vi "picture plot.vi"(8 "error in":errorcluster) -> (0 "error out":errorcluster, 3 "Images":picture[](array[picture]))   [LabVIEW 2018]
uses:
  channel_cluster.ctl
  <vilib>/picture/cartesn2.llb/XY Plot Type.ctl
  CAEN globals.vi
panel:
  out "new picture":picture
  # "mrd1\nmrd2\ntank\nveto\nother\nmaster"
  # "mrd1 = pink\nmrd2 = green\ntank = blue\nveto = orange\nmasters = purple\nother = red"
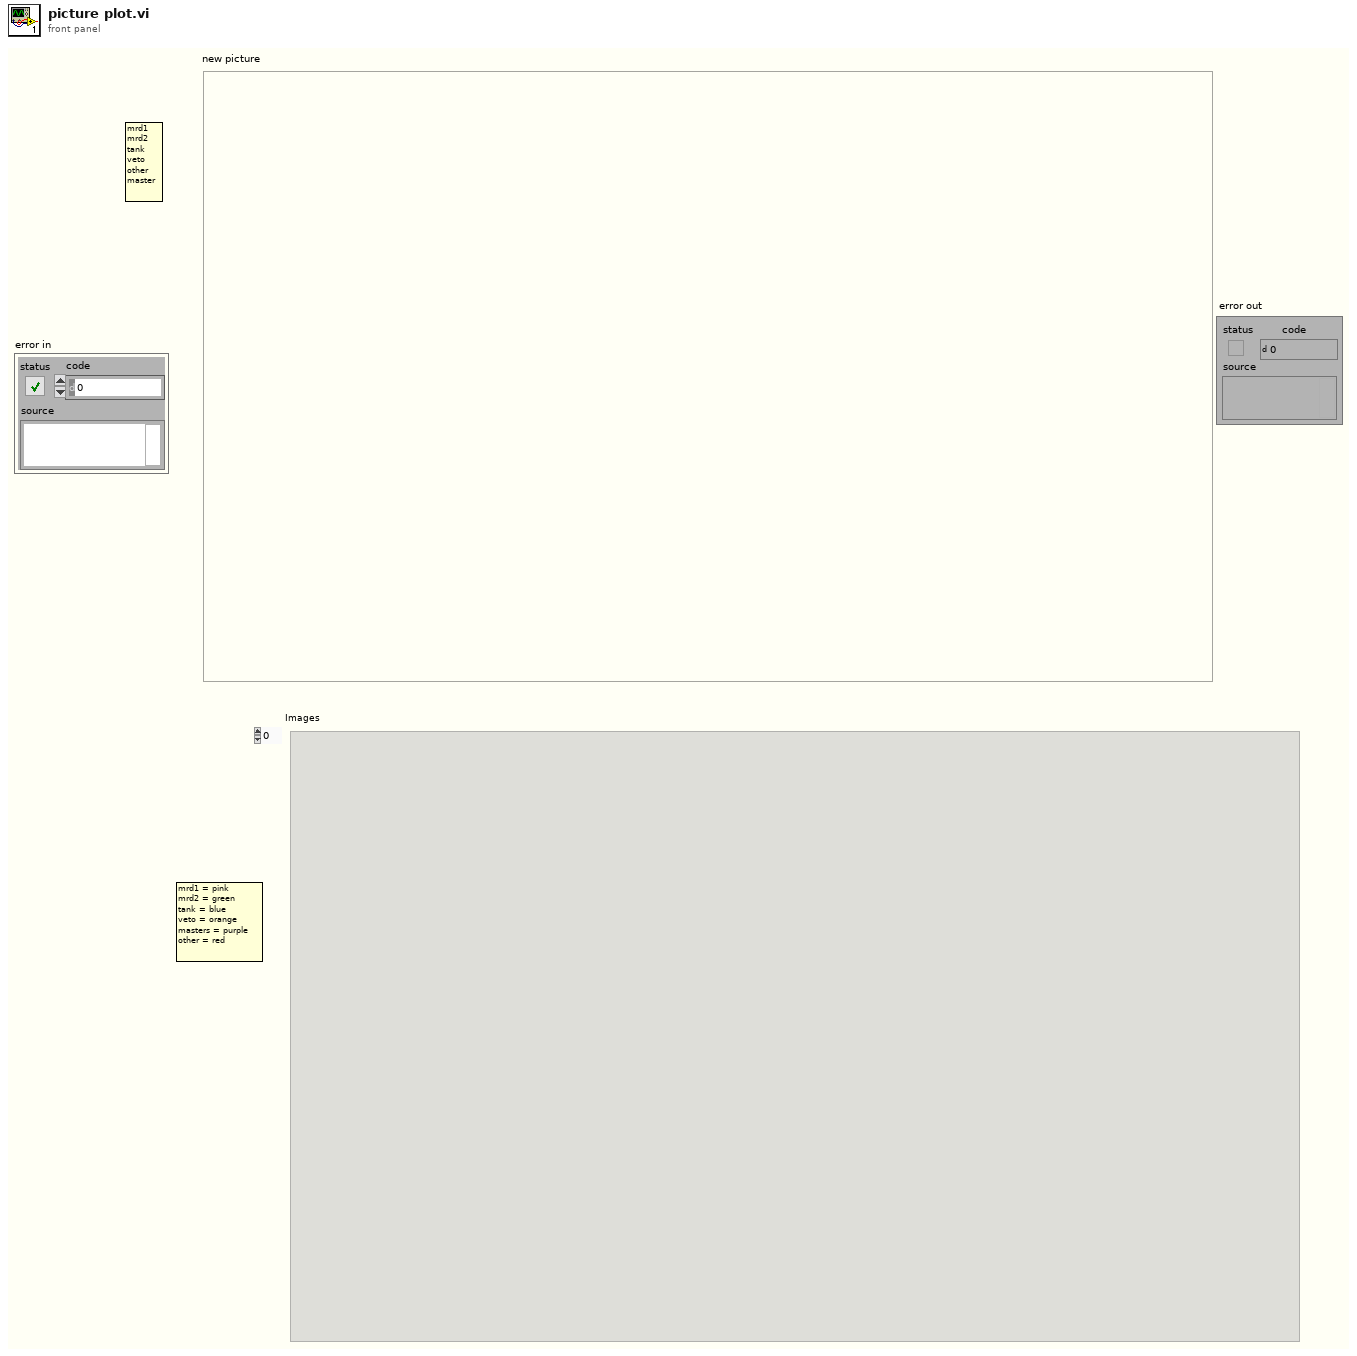
[diagram p1: front panel]
types:
  T1 = typedef "channel_cluster.ctl" = cluster{"Channel Name":string, "Crate":i32, "Card Type":string, "Card":i32, "Channel":i32, "Status Icon":picture, "Vmon (V)":dbl, "Vset (V)":dbl, "Imon (A)":dbl, "Iset (A)":dbl, "Timestamp":string, "ON/OFF":bool, "Status":string, "Vswmax (V)":dbl, "Flag":bool, "Vfile (V)":dbl, "Error Logged":bool[], "enable_file":bool}
  T2 = cluster{"x minimum":dbl, "x maximum":dbl, "x log?":bool, "x precision":u8, "x format":enum8{"Decimal", "Scientific", "Engineering", "Binary", "Octal", "Hex", "Timestamp"}, "y minimum":dbl, "y maximum":dbl, "y log?":bool, "y precision":u8, "y format":enum8{"Decimal", "Scientific", "Engineering", "Binary", "Octal", "Hex", "Timestamp"}}
  T3 = cluster{"Width":u16, "Style":enum32{"Solid", "Dash", "Dot", "DashDot", "DashDotDot"}}[]
  T4 = enum8{"Decimal", "Scientific", "Engineering", "Binary", "Octal", "Hex", "Timestamp"}
  T5 = typedef "XY Plot Type.ctl" = enum16{"points", "squares", "circles", "connected points", "connected squares", "connected circles", "comb plot", "sized scatter plot", "sized-colored scatter plot", "min-max lines"}
  T6 = cluster{"plot color":u32, "XY plot type":T5, "baseline":dbl}
  T7 = cluster{"line color":u32, "text color":u32, "tick length(3)":i16, "crossing axes":bool, "visible grid?":bool}
  T8 = cluster{"plot color":u32, "XY plot type":T5, "baseline":dbl}[]
  T9 = typedef "imagedata.ctl" = cluster{"image type":i32, "image depth":i32, "image":u8[], "mask":u8[], "colors":u32[], "Rectangle":cluster{"left":i16, "top":i16, "right":i16, "bottom":i16}}
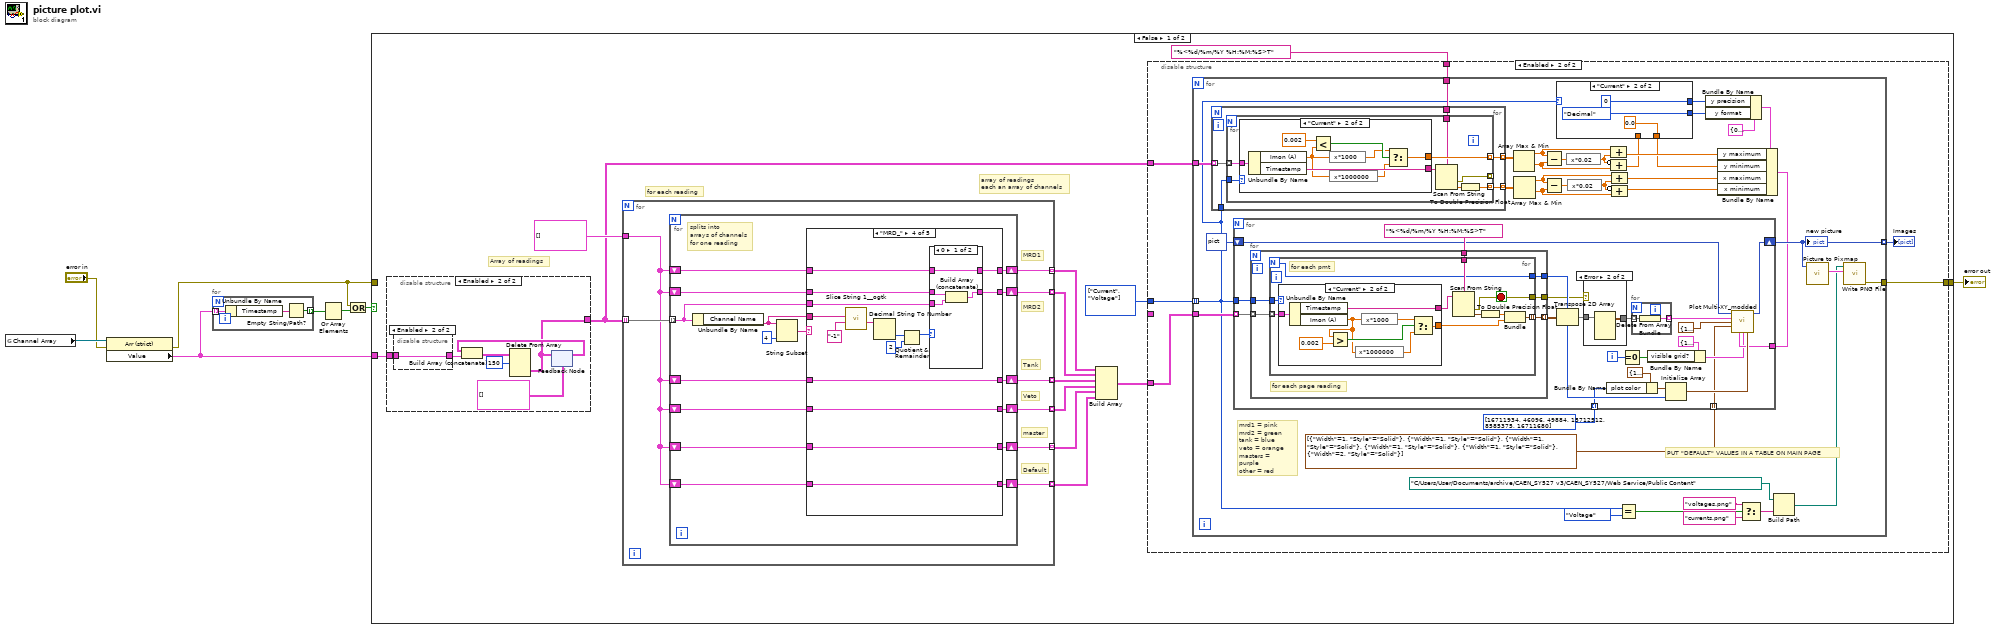
[diagram p0: block diagram]
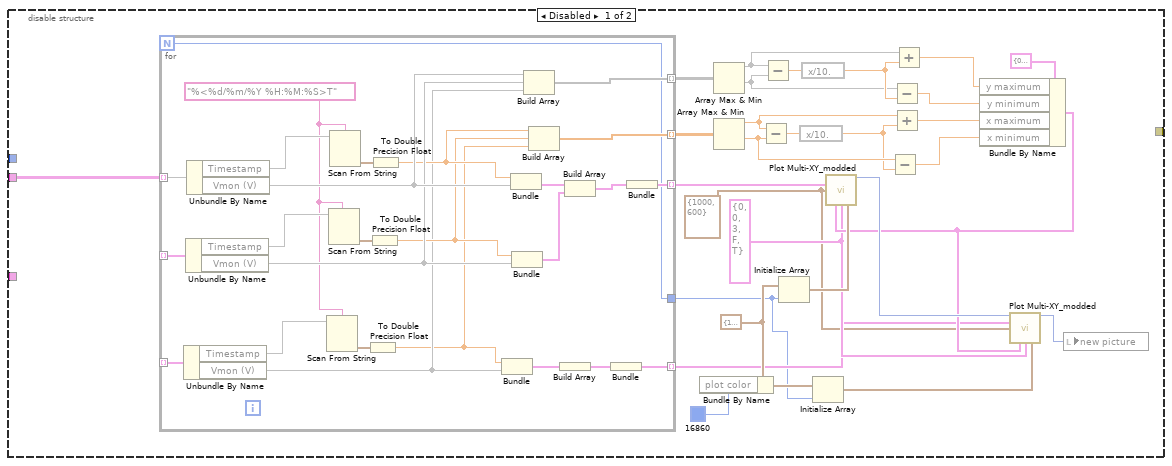
[diagram p4: hidden frame]
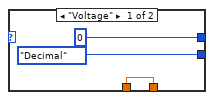
[diagram p5: hidden frame]
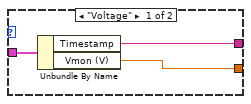
[diagram p7: hidden frame]
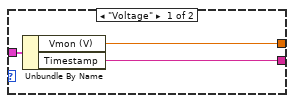
[diagram p8: hidden frame]
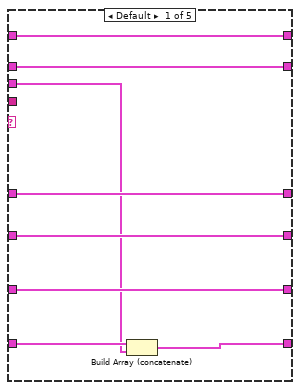
[diagram p9: hidden frame]
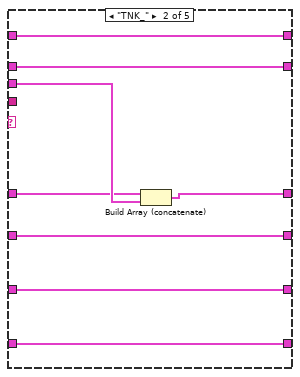
[diagram p10: hidden frame]
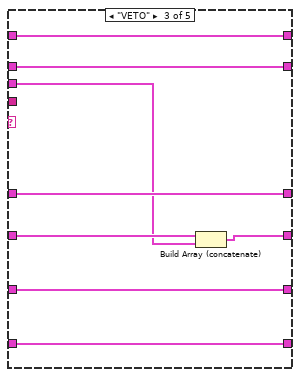
[diagram p11: hidden frame]
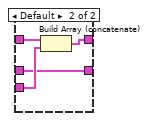
[diagram p12: hidden frame]
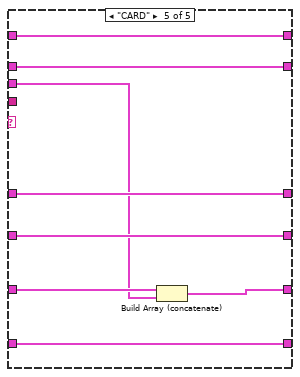
[diagram p13: hidden frame]
diagram:
  n1 = global read "CAEN globals.vi" "Channel Array"() -> (w7:refnum<vi>)
  n2 = property class="Arr (strict)"(reference=w7, error in="error in") -> (error out=w3:errorcluster, "Value"=w5:T1[])  [unwired: 1 out]
  n3 = for {
    tunnel: w5 -> [w11] mode=indexing
    tunnel: [w9] -> w4 mode=indexing
    n4 = Unbundle By Name(w11) -> ("Timestamp"=w10:string)
    n5 = Empty String/Path?(string/path=w10) -> (empty?=w9:bool)
  }
  n6 = Or Array Elements(Boolean array=w4) -> (logical OR=w2:bool)
  n7 = Or(x=w3, y=w2) -> (x .or. y?=w1:bool)
  n8 = case shown="False" w1 {
    tunnel: [w15 w294] -> w8
    tunnel: w5 -> [w12 _]
    tunnel: w3 -> [_ w294]
    frame False {
      w14 = enum16{"Current", "Voltage"}[] [enum."Current", enum."Voltage"] items=["Current", "Voltage"]
      # "array of readings\neach an array of channels"
      # "for each reading"
      # "Array of readings"
      n9 = disable-structure shown="Enabled" {
        disable-tunnel: [_ w27] -> w18
        disable-tunnel: w12 -> [_ w25]
        frame Disabled {
        }
        frame Enabled {
          n10 = disable-structure shown="Enabled" {
            disable-tunnel: [_ w32] -> w29
            disable-tunnel: w25 -> [_ w32]
            frame Disabled {
            }
            frame Enabled {
            }
          }
          n11 = feedback #1(T1[][] [] ("appended array")) -> (w30:T1[][])
          n12 = Build Array (concatenate)(w30, w29) -> (w28:T1[][])
          n13 = Delete From Array(array=w28, length=150) -> (deleted portion=w27:T1[][])  [unwired: 2 in, 1 out]
          n14 = feedback-in #1(w27) -> ()
        }
      }
      n15 = for {
        tunnel: w18 -> [w222] mode=indexing
        tunnel: [w221] -> w19 mode=indexing
        tunnel: [w220] -> w23 mode=indexing
        tunnel: [w219] -> w16 mode=indexing
        tunnel: [w218] -> w22 mode=indexing
        tunnel: [w217] -> w21 mode=indexing
        tunnel: T1[] [] -> [w216]
        tunnel: [w215] -> w13 mode=indexing
        # "master"
        # "Default"
        # "Veto"
        # "Tank"
        # "MRD2"
        # "MRD1"
        n16 = for {
          shift-right: [w232] -> w218
          shift-left: w216 -> [w231]
          shift-right: [w234] -> w219
          shift-left: w216 -> [w233]
          shift-right: [w228] -> w220
          shift-left: w216 -> [w235]
          shift-right: [w229] -> w221
          shift-left: w216 -> [w236]
          tunnel: w222 -> [w230] mode=indexing
          shift-right: [w227] -> w217
          shift-left: w216 -> [w226]
          shift-right: [w223] -> w215
          shift-left: w216 -> [w224]
          # "splits into \narrays of channels\nfor one reading"
          n17 = Unbundle By Name(w230) -> ("Channel Name"=w225:string)
          n18 = String Subset(string=w225, length (rest)=4 ("length (rest)")) -> (substring=w237:string)  [unwired: 1 in]
          n19 = case shown="\"MRD_\"" w237 {
            tunnel: w236 -> [w246 w254 w262 w272 w293]
            tunnel: w235 -> [w245 w253 w261 w268 w292]
            tunnel: [w244 w250 w260 w274 w291] -> w234
            tunnel: w233 -> [w244 w251 w260 w274 w291]
            tunnel: [w243 w249 w257 w273 w290] -> w232
            tunnel: w231 -> [w243 w249 w259 w273 w290]
            tunnel: w230 -> [w239 w252 w258 w271 w288]
            tunnel: [w246 w254 w262 w270 w293] -> w229
            tunnel: [w245 w253 w261 w269 w292] -> w228
            tunnel: [w242 w248 w256 w267 w287] -> w227
            tunnel: w226 -> [w242 w248 w256 w267 w289]
            tunnel: w225 -> [_ _ _ w266 _]
            tunnel: w224 -> [w241 w247 w255 w263 w286]
            tunnel: [w240 w247 w255 w263 w286] -> w223
            frame Default {
              n20 = Build Array (concatenate)(w241, w239) -> (w240:T1[])
            }
            frame "TNK_" {
              n21 = Build Array (concatenate)(w251, w252) -> (w250:T1[])
            }
            frame "VETO" {
              n22 = Build Array (concatenate)(w259, w258) -> (w257:T1[])
            }
            frame "MRD_" {
              n23 = call <userlib>:"Slice String 1__ogtk.vi"("Subset (i:j)"="-1", "String"=w266) -> ("Substring (String[i:j])"=w277:string)  [unwired: 7 in]
              n24 = Decimal String To Number(string=w277) -> (number=w276:i32)  [unwired: 2 in, 1 out]
              n25 = Quotient & Remainder(x=w276, y=2) -> (x-y*floor(x/y)=w265:i32)  [unwired: 1 out]
              n26 = case shown="0" w265 {
                tunnel: w272 -> [w281 w285]
                tunnel: w271 -> [w278 w284]
                tunnel: [w281 w283] -> w270
                tunnel: [w279 w282] -> w269
                tunnel: w268 -> [w280 w282]
                frame 0 {
                  n27 = Build Array (concatenate)(w280, w278) -> (w279:T1[])
                }
                frame Default {
                  n28 = Build Array (concatenate)(w285, w284) -> (w283:T1[])
                }
              }
            }
            frame "CARD" {
              n29 = Build Array (concatenate)(w289, w288) -> (w287:T1[])
            }
          }
        }
      }
      n30 = Build Array(w19, w23, w16, w22, w21, w13) -> (w20:T1[][][])
      n31 = disable-structure shown="Enabled" {
        disable-tunnel: _ -> [w34 _]
        disable-tunnel: w20 -> [_ w91]
        disable-tunnel: w18 -> [_ w93]
        disable-tunnel: "%<%d/%m/%Y %H:%M:%S>T" ("format string") -> [_ w92]
        disable-tunnel: [_ w90] -> w15
        disable-tunnel: w14 -> [_ w88]
        frame Disabled {
          w41 = T6 {"plot color"=16711680, "XY plot type"=enum."connected points", "baseline"=0.0} ("xy plot cosmetics")
          w42 = T7 {"line color"=0, "text color"=0, "tick length(3)"=3, "crossing axes"=FALSE, "visible grid?"=TRUE} ("cartesian grid cosmetics")
          w38 = cluster{"width":i16, "height":i16} {"width"=1000, "height"=600} ("dimensions (w,h)")
          n32 = for {
            N -> [w75]
            tunnel: w34 -> [w87] mode=indexing
            tunnel: [w82] -> w61 mode=indexing
            tunnel: [w76] -> w60 mode=indexing
            tunnel: [w77] -> w54 mode=indexing
            tunnel: _ -> [w79] mode=indexing
            tunnel: [w75] -> w35
            tunnel: _ -> [w68] mode=indexing
            tunnel: [w64] -> w39 mode=indexing
            w67 = "%<%d/%m/%Y %H:%M:%S>T" ("format string")
            n33 = Unbundle By Name(w68) -> ("Timestamp"=w70, "Vmon (V)"=w63)
            n34 = Unbundle By Name(w79) -> ("Timestamp"=w80, "Vmon (V)"=w73)
            n35 = Unbundle By Name(w87) -> ("Timestamp"=w86, "Vmon (V)"=w74)
            n36 = Scan From String(format string=w67, input string=w70) -> (output 1=w69:timestamp)  [unwired: 3 in, 3 out]
            n37 = Scan From String(format string=w67, input string=w80) -> (output 1=w81:timestamp)  [unwired: 3 in, 3 out]
            n38 = Scan From String(format string=w67, input string=w86) -> (output 1=w85:timestamp)  [unwired: 3 in, 3 out]
            n39 = To Double Precision Float(number=w69) -> (double precision float=w62:dbl)
            n40 = To Double Precision Float(number=w81) -> (double precision float=w71:dbl)
            n41 = To Double Precision Float(number=w85) -> (double precision float=w72:dbl)
            n42 = Bundle(w62, "Vmon (V)"=w63) -> (w66:cluster{dbl, "Vmon (V)":void})  [unwired: 1 in]
            n43 = Bundle(w72, "Vmon (V)"=w74) -> (w84:cluster{dbl, "Vmon (V)":void})  [unwired: 1 in]
            n44 = Bundle(w71, "Vmon (V)"=w73) -> (w78:cluster{dbl, "Vmon (V)":void})  [unwired: 1 in]
            n45 = Build Array(w74, w73, w63) -> (w77:void[])
            n46 = Build Array(w72, w71, w62) -> (w76:dbl[])
            n47 = Build Array(w66) -> (w65:cluster{dbl, "Vmon (V)":void}[])
            n48 = Build Array(w84, w78) -> (w83:cluster{dbl, "Vmon (V)":void}[])
            n49 = Bundle(w65) -> (w64:cluster{cluster{dbl, "Vmon (V)":void}[]})  [unwired: 1 in]
            n50 = Bundle(w83) -> (w82:cluster{cluster{dbl, "Vmon (V)":void}[]})  [unwired: 1 in]
          }
          n51 = Bundle By Name(cluster=w41, "plot color"=u32 16860) -> (w37:T6)
          n52 = Array Max & Min(array=w54) -> (max value=w49, min value=w48)  [unwired: 2 out]
          n53 = Array Max & Min(array=w60) -> (max value=w58:dbl, min value=w57:dbl)  [unwired: 2 out]
          n54 = Subtract(x=w58, y=w57) -> (x-y=w59:dbl)
          n55 = Subtract(x=w49, y=w48) -> (x-y=w50:dbl)
          n56 = Initialize Array(w41, w35) -> (w45:T8)
          n57 = expression code="x/10."(w59) -> (w56:dbl)
          n58 = expression code="x/10."(w50) -> (w51:dbl)
          n59 = Initialize Array(w37, w35) -> (w36:T8)
          n60 = Subtract(x=w57, y=w56) -> (x-y=w52:dbl)
          n61 = Subtract(x=w48, y=w51) -> (x-y=w46:dbl)
          n62 = Add(x=w58, y=w56) -> (x+y=w53:dbl)
          n63 = Add(x=w49, y=w51) -> (x+y=w47:dbl)
          n64 = Bundle By Name(cluster=T2 {"x minimum"=0.0, "x maximum"=0.0, "x log?"=FALSE, "x precision"=2, "x format"=enum."Timestamp", "y minimum"=0.0, "y maximum"=0.0, "y log?"=FALSE, "y precision"=0, "y format"=enum."Decimal"} ("cartesian axis attributes"), "y maximum"=w47, "y minimum"=w46, "x maximum"=w53, "x minimum"=w52) -> (w43:T2)
          n65 = call "Plot Multi-XY_modded.vi"("data"=w61, "dimensions (w,h)"=w38, "cartesian axis attributes"=w43, "cartesian grid cosmetics"=w42, "XY plot cosmetics"=w45) -> ("new picture"=w44:picture)  [unwired: 10 in]
          n66 = call "Plot Multi-XY_modded.vi"("picture"=w44, "data"=w39, "dimensions (w,h)"=w38, "cartesian axis attributes"=w43, "cartesian grid cosmetics"=w42, "XY plot cosmetics"=w36) -> ("new picture"=w33:picture)  [unwired: 9 in]
          n67 = local write "new picture"(w33) -> ()
        }
        frame Enabled {
          n68 = for {
            tunnel: w93 -> [w124]
            tunnel: w92 -> [w123]
            tunnel: w91 -> [w121]
            tunnel: [w117] -> w90
            tunnel: [w109] -> w89 mode=indexing
            tunnel: w88 -> [w105] mode=indexing
            # "PUT \"DEFAULT\" VALUES IN A TABLE ON MAIN PAGE"
            # "mrd1 = pink\nmrd2 = green\ntank = blue\nveto = orange\nmasters = purple\nother = red"
            n69 = for {
              tunnel: w124 -> [w195] mode=indexing
              tunnel: [w194] -> w96 mode=indexing
              tunnel: w123 -> [w193]
              tunnel: [w192] -> w122 mode=indexing
              tunnel: w105 -> [w191]
              n70 = for {
                tunnel: w195 -> [w203] mode=indexing
                tunnel: [w202] -> w194 mode=indexing
                tunnel: w193 -> [w199]
                tunnel: [w198] -> w192 mode=indexing
                tunnel: w191 -> [w197]
                tunnel: [w196] -> _ mode=indexing
                n71 = case shown="\"Current\"" w197 {
                  tunnel: w203 -> [w206 w214]
                  tunnel: [w205 w211] -> w202
                  tunnel: [w204 w213] -> w200
                  frame "Voltage" {
                    n72 = Unbundle By Name(w206) -> ("Vmon (V)"=w205:dbl, "Timestamp"=w204:string)
                  }
                  frame "Current" {
                    n73 = Unbundle By Name(w214) -> ("Imon (A)"=w210:dbl, "Timestamp"=w213:string)
                    n74 = Less?(x=0.002, y=w210) -> (x < y?=w209:bool)
                    n75 = expression code="x*1000"(w210) -> (w208:dbl)
                    n76 = expression code="x*1000000"(w210) -> (w207:dbl)
                    n77 = Select(t=w208, s=w209, f=w207) -> (s? t:f=w211:dbl)
                  }
                }
                n78 = Scan From String(format string=w199, input string=w200) -> (error out=w196:errorcluster, output 1=w201:dbl)  [unwired: 3 in, 2 out]
                n79 = To Double Precision Float(number=w201) -> (double precision float=w198:dbl)
              }
            }
            n80 = Array Max & Min(array=w96) -> (max value=w99:dbl, min value=w100:dbl)  [unwired: 2 out]
            n81 = Array Max & Min(array=w122) -> (max value=w129:dbl, min value=w128:dbl)  [unwired: 2 out]
            n82 = Subtract(x=w99, y=w100) -> (x-y=w98:dbl)
            n83 = Subtract(x=w129, y=w128) -> (x-y=w130:dbl)
            n84 = expression code="x*0.02"(w98) -> (w101:dbl)
            n85 = expression code="x*0.02"(w130) -> (w127:dbl)
            n86 = Compound Arithmetic op=ADD(w99, w101) -> (w97:dbl)
            n87 = Compound Arithmetic op=ADD(invert w101, w100) -> (w95:dbl)
            n88 = case shown="\"Current\"" w105 {
              tunnel: [u8 0 ("y precision") u8 0 ("y precision")] -> w104
              tunnel: [T4."Decimal" ("y format") T4."Decimal" ("y format")] -> w103
              tunnel: [w131 0.0] -> w94
              tunnel: w95 -> [w131 _]
              frame "Voltage" {
              }
              frame "Current" {
              }
            }
            n89 = Compound Arithmetic op=ADD(w129, w127) -> (w126:dbl)
            n90 = Compound Arithmetic op=ADD(invert w127, w128) -> (w125:dbl)
            n91 = Equal?(x=w105, y=enum16{"Current", "Voltage"}."Voltage") -> (x = y?=w111:bool)
            n92 = Bundle By Name(cluster=T2 {"x minimum"=0.0, "x maximum"=0.0, "x log?"=FALSE, "x precision"=2, "x format"=enum."Timestamp", "y minimum"=0.0, "y maximum"=0.0, "y log?"=FALSE, "y precision"=0, "y format"=enum."Decimal"} ("cartesian axis attributes"), "y precision"=w104, "y format"=w103) -> (w106:T2)
            n93 = Bundle By Name(cluster=w106, "y maximum"=w97, "y minimum"=w94, "x maximum"=w126, "x minimum"=w125) -> (w102:T2)
            n94 = for {
              tunnel: w102 -> [w157]
              tunnel: w121 -> [w143] mode=indexing
              tunnel: u32[] [16711934, 46096, 49884, 15712512, 8585375, 16711680] -> [w151] mode=indexing
              shift-right: [w150] -> w109
              shift-left: picture data[5B] ("new picture") -> [w149]
              tunnel: T3 [{"Width"=1, "Style"=enum."Solid"}, {"Width"=1, "Style"=enum."Solid"}, {"Width"=1, "Style"=enum."Solid"}, {"Width"=1, "Style"=enum."Solid"}, {"Width"=1, "Style"=enum."Solid"}, {"Width"=2, "Style"=enum."Solid"}] -> [w138] mode=indexing
              tunnel: w105 -> [w137]
              i -> [w140]
              n95 = for {
                tunnel: w143 -> [w169] mode=indexing
                tunnel: [w165] -> w155
                tunnel: "%<%d/%m/%Y %H:%M:%S>T" ("format string") -> [w168]
                tunnel: [w167] -> w145 mode=indexing
                tunnel: [w166] -> w144
                tunnel: w137 -> [w164]
                # "for each page reading"
                n96 = for {
                  N -> [w171]
                  tunnel: w169 -> [w179] mode=indexing
                  tunnel: [w174] -> w167 mode=indexing
                  tunnel: w168 -> [w173]
                  tunnel: [w172] -> w166
                  tunnel: [w171] -> w165
                  tunnel: w164 -> [w170]
                  stop <- w172 stop-if-true
                  # "for each pmt"
                  n97 = case shown="\"Current\"" w170 {
                    tunnel: w179 -> [w182 w190]
                    tunnel: [w181 w189] -> w178
                    tunnel: [w180 w184] -> w176
                    frame "Voltage" {
                      n98 = Unbundle By Name(w182) -> ("Timestamp"=w181:string, "Vmon (V)"=w180:dbl)
                    }
                    frame "Current" {
                      n99 = Unbundle By Name(w190) -> ("Timestamp"=w189:string, "Imon (A)"=w183:dbl)
                      n100 = Greater?(x=w183, y=0.002 ("x")) -> (0:w186:bool)
                      n101 = expression code="x*1000000"(w183) -> (w188:dbl)
                      n102 = expression code="x*1000"(w183) -> (w187:dbl)
                      n103 = Select(t=w187, s=w186, f=w188) -> (s? t:f=w184:dbl)
                    }
                  }
                  n104 = Scan From String(format string=w173, input string=w178) -> (error out=w172:errorcluster, output 1=w177:timestamp)  [unwired: 3 in, 2 out]
                  n105 = To Double Precision Float(number=w177) -> (double precision float=w175:dbl)
                  n106 = Bundle(w175, "Imon (A)"=w176) -> (w174:cluster{dbl, "Imon (A)":dbl})  [unwired: 1 in]
                }
              }
              n107 = Transpose 2D Array(2D array=w145) -> (transposed array=w148:cluster{dbl, "Imon (A)":dbl}[][])
              n108 = case shown="Error" w144 {
                tunnel: w148 -> [w159 w161]
                tunnel: [w159 w160] -> w147
                frame No Error {
                }
                frame Error {
                  n109 = Delete From Array(array=w161) -> (array with subset deleted=w160:cluster{dbl, "Imon (A)":dbl}[][])  [unwired: 3 in, 1 out]
                }
              }
              n110 = Bundle By Name(cluster=T6 {"plot color"=16711680, "XY plot type"=enum."connected circles", "baseline"=0.0} ("xy plot cosmetics"), "plot color"=w151) -> (w152:T6)
              n111 = Equal To 0?(x=w140) -> (x = 0?=w139:bool)
              n112 = for {
                tunnel: w147 -> [w163] mode=indexing
                tunnel: [w162] -> w146 mode=indexing
                n113 = Bundle(w163) -> (w162:cluster{cluster{dbl, "Imon (A)":dbl}[]})  [unwired: 1 in]
              }
              n114 = Bundle By Name(cluster=T7 {"line color"=13816530, "text color"=0, "tick length(3)"=3, "crossing axes"=FALSE, "visible grid?"=TRUE} ("cartesian grid cosmetics"), "visible grid?"=w139) -> (w141:T7)
              n115 = Initialize Array(w152, w155) -> (w158:T8)
              n116 = call "Plot Multi-XY_modded.vi"("picture"=w149, "data"=w146, "dimensions (w,h)"=cluster{"width":i16, "height":i16} {"width"=1000, "height"=600}, "line style"=w138, "cartesian axis attributes"=w157, "cartesian grid cosmetics"=w141, "XY plot cosmetics"=w158) -> ("new picture"=w150:picture)  [unwired: 8 in]
            }
            "new picture" <- w109
            n117 = Select(t="voltages.png" ("name or relative path"), s=w111, f="currents.png" ("name or relative path")) -> (s? t:f=w113:string)
            n118 = Build Path(base path=path "C:/Users/User/Documents/archive/CAEN_SY527 v3/CAEN_SY527/Web Service/Public Content" ("FIle to save"), name or relative path=w113) -> (appended path=w115:path)
            n119 = call <vilib>:"Picture to Pixmap.vi"("picture"=w109) -> ("image data"=w118:T9)  [unwired: 9 in, 1 out]
            n120 = call <vilib>:"Write PNG File.vi"("image data"=w118, "path to PNG file"=w115) -> ("error out"=w117:errorcluster)  [unwired: 8 in, 1 out]
          }
          "Images" <- w89
        }
      }
    }
    frame True {
    }
  }
  "error out" <- w8
